vi "cRIO_ZNB_AMI_GLOBALES.vi"() -> ()   [LabVIEW 2017]
uses:
  RohdeSchwarz ZNB MeasConfig.ctl
  AMI MAGNET/Status AMI.ctl
  WEB Readings/Temperaturas Bluefors.ctl
  AMI MAGNET/commsControl.ctl
panel:
  in  "EN":bool
  in  "x":dbl min=-0.5 max=0.5 step=0.001 format="%.2f"
  in  "y":dbl min=-0.5 max=0.5 step=0.001 format="%.2f"
  out "ConfigX":T1={"connection ID"=refnum, "IP"="192.168.0.108", "Active Comm Interface"=0, "Serial Port"="", "Programmer Type"=0, "connection ID"=refnum, "output cluster"={"GPIB address"=22, "GPIB bus"=1}} {"Programmer Type" items=["Model 430", "Model 420"]; "Active Comm Interface" items=["TCP/IP (Model 430 Only)", "RS232", "IEEE488"]}
  out "ConfigY":T1={"connection ID"=refnum, "IP"="192.168.0.108", "Active Comm Interface"=0, "Serial Port"="", "Programmer Type"=0, "connection ID"=refnum, "output cluster"={"GPIB address"=22, "GPIB bus"=1}} {"Programmer Type" items=["Model 430", "Model 420"]; "Active Comm Interface" items=["TCP/IP (Model 430 Only)", "RS232", "IEEE488"]}
  out "ConfigZ":T1={"connection ID"=refnum, "IP"="192.168.0.108", "Active Comm Interface"=0, "Serial Port"="", "Programmer Type"=0, "connection ID"=refnum, "output cluster"={"GPIB address"=22, "GPIB bus"=1}} {"Programmer Type" items=["Model 430", "Model 420"]; "Active Comm Interface" items=["TCP/IP (Model 430 Only)", "RS232", "IEEE488"]}
  in  "Remote GO XYZ":bool
  out "F Stable":bool
  in  "FRemoteChange":bool
  out "Field Status":i32(ring) items=["MagnetUnknown"=0, "StablePersistent"=1, "WarmingSwitch"=2, "CoolingSwitch"=3, "StableDriven"=4, "Iterating"=5, "Charging"=6, "Discharging"=7, "CurrentError"=8, "MagnetFailure"=15]
  in  "MagneticField(T)":dbl
  in  "R_spField(T)":dbl=20.0
  in  "W_spField(T)":dbl
  in  "Rate(T/min)":dbl=0.1
  in  "SetpointB(T)":dbl
  in  "Electroiman(s)":dbl=0.5
  in  "ElectroimanEnable":bool=TRUE
  in  "stopElectroiman":bool
  in  "Remote DEMAG X":bool
  in  "Remote DEMAG Y":bool
  in  "Remote DEMAG Z":bool
  out "Z Stable":bool
  out "Y Stable":bool
  in  "BF RemoteChange":bool
  in  "url":string="http://192.168.0.101:5001/channel/measurement/latest"
  in  "Enable BF(T)":bool=TRUE
  in  "stopBluefors":bool
  out "BLUEFORS":T2 {"Canal 8" format="%.3f"; "Canal 7" format="%.3f"; "Canal 6" format="%.3f"; "Canal 5" format="%.3f"; "Canal 4" format="%.3f"; "Canal 3" format="%.3f"; "Canal 2" format="%.3f"; "Canal 1" format="%.3f"}
  in  "rampingMode X":u16(ring)=1 items=["RAMP", "PAUSE", "MANUAL UP", "MANUAL DOWN", "ZERO"]
  in  "rampingMode Y":u16(ring)=1 items=["RAMP", "PAUSE", "MANUAL UP", "MANUAL DOWN", "ZERO"]
  in  "rampingMode Z":u16(ring)=1 items=["RAMP", "PAUSE", "MANUAL UP", "MANUAL DOWN", "ZERO"]
  in  "stopMagneticField":bool
  in  "Remote SET Z":bool
  in  "Remote GO X":bool
  in  "Remote GO Y":bool
  in  "Remote SET X":bool
  in  "Remote SET Y":bool
  in  "Remote GO Z":bool
  out "X state":T3=1 items=["Unknown", "RAMPING to target field/current", "HOLDING at the target field/current", "PAUSED", "Ramping in MANUAL UP mode", "Ramping in MANUAL DOWN mode", "ZEROING CURRENT (in progress)", "Quench detected", "At ZERO current", "Heating persistent switch", "Cooling persistent switch", "External Rampdown active"]
  in  "Target X":dbl format="%.2f"
  in  "Rate X":dbl=0.1 format="%.2f"
  out "X field":dbl format="%.2f"
  out "Y state":T3=1 items=["Unknown", "RAMPING to target field/current", "HOLDING at the target field/current", "PAUSED", "Ramping in MANUAL UP mode", "Ramping in MANUAL DOWN mode", "ZEROING CURRENT (in progress)", "Quench detected", "At ZERO current", "Heating persistent switch", "Cooling persistent switch", "External Rampdown active"]
  in  "Target Y":dbl format="%.2f"
  in  "Rate Y":dbl=0.1 format="%.2f"
  out "Y field":dbl format="%.2f"
  out "Z state":T3=1 items=["Unknown", "RAMPING to target field/current", "HOLDING at the target field/current", "PAUSED", "Ramping in MANUAL UP mode", "Ramping in MANUAL DOWN mode", "ZEROING CURRENT (in progress)", "Quench detected", "At ZERO current", "Heating persistent switch", "Cooling persistent switch", "External Rampdown active"]
  in  "Target Z":dbl format="%.2f"
  in  "Rate Z":dbl=0.1 format="%.2f"
  out "Z field":dbl format="%.2f"
  out "Z ramping":bool
  out "Y ramping":bool
  out "X ramping":bool
  out "XY Graph":cluster{dbl[], dbl[]}(graph)
  out "VISA ENA3G":refnum<visa-resource-name>="GPIB0::17::INSTR"
  in  "ENA3G Config":T4={"Tiempo (sec)"=10.0, "Campo X (T)"=0.025, "Campo Y (T)"=10.0, "Campo Z (T)"=0.025, "Temperatura (K)"=0.025, "Start Frequency (Hz)"=100000.0, "Stop Frequency (Hz)"=1000000.0, "IF Bandwidth"=25.0, "Sweep time(s)"=25.0, "Meas Points"=201, "Power Level (0.0)"=-40.0} {"Campo Z (T)" format="%^.2e"; "Campo Y (T)" format="%^.2e"; "Sweep time(s)" format="%^.2g"; "Temperatura (K)" format="%^.2e"; "Campo X (T)" format="%^.2e"; "Tiempo (sec)" format="%^.2g"; "Start Frequency (Hz)" format="%^.2e"; "IF Bandwidth" format="%^.2e"; "Power Level (0.0)" format="%^.2g"}
  in  "VRemoteChange":bool
  out "Voltage Status":i32(ring) items=["VoltageUnknown", "Stable", "Tracking"]
  out "V Stable":bool
  in  "RampaVolt(V)":dbl
  in  "R_spVolt(V)":dbl=20.0
  in  "W_spVolt(V)":dbl
  in  "Rate(V/min)":dbl=0.1
  in  "SetpointV(V)":dbl
  in  "RampaVolt(s)":dbl=0.5
  in  "RampaVoltajeEnable":bool=TRUE
  in  "stopRampaVolt":bool
  in  "FieldCalPath":path=path "C:/Users/pemar/Documents/LabVIEW Data/XImanCalibre.txt"
  in  "TempCalPath":path=path "C:/Users/pemar/Documents/LabVIEW Data/X71548_InterpNew.txt"
  in  "TRemoteChange":bool
  out "DataPath":path
  out "Total Comandos":i32
  out "Comando actual":i32
  out "TotalSequence":string[](array[string])
  in  "stop":bool
  out "Temperature Status":i32(ring) items=["TemperatureUnknown", "Stable", "Tracking", "Near"]
  out "X Stable":bool
  out "T Stable":bool
  in  "R_spTemp(K)":dbl=20.0
  in  "W_spTemp(K)":dbl
  in  "VISA LakeShore":refnum<visa-resource-name>="COM3"
  in  "SaveData":bool=TRUE
  in  "Rate(K/min)":dbl=20.0
  in  "SetpointT(K)":dbl
  in  "Temperatura(K)":dbl
  in  "LakeShoreEnable":bool=TRUE
  in  "LakeShore(s)":dbl=0.5
  in  "stopLakeShore":bool
  in  "Estado":bool=TRUE
  in  "InitGraph":bool=TRUE
  in  "AMI Enable":bool=TRUE
  # "Z axis"
  # "Y axis"
  # "X axis"
  # "STATUS"
  # "STATUS"
  # "STATUS"
  # "SETTINGS"
  # "SETTINGS"
  # "SETTINGS"
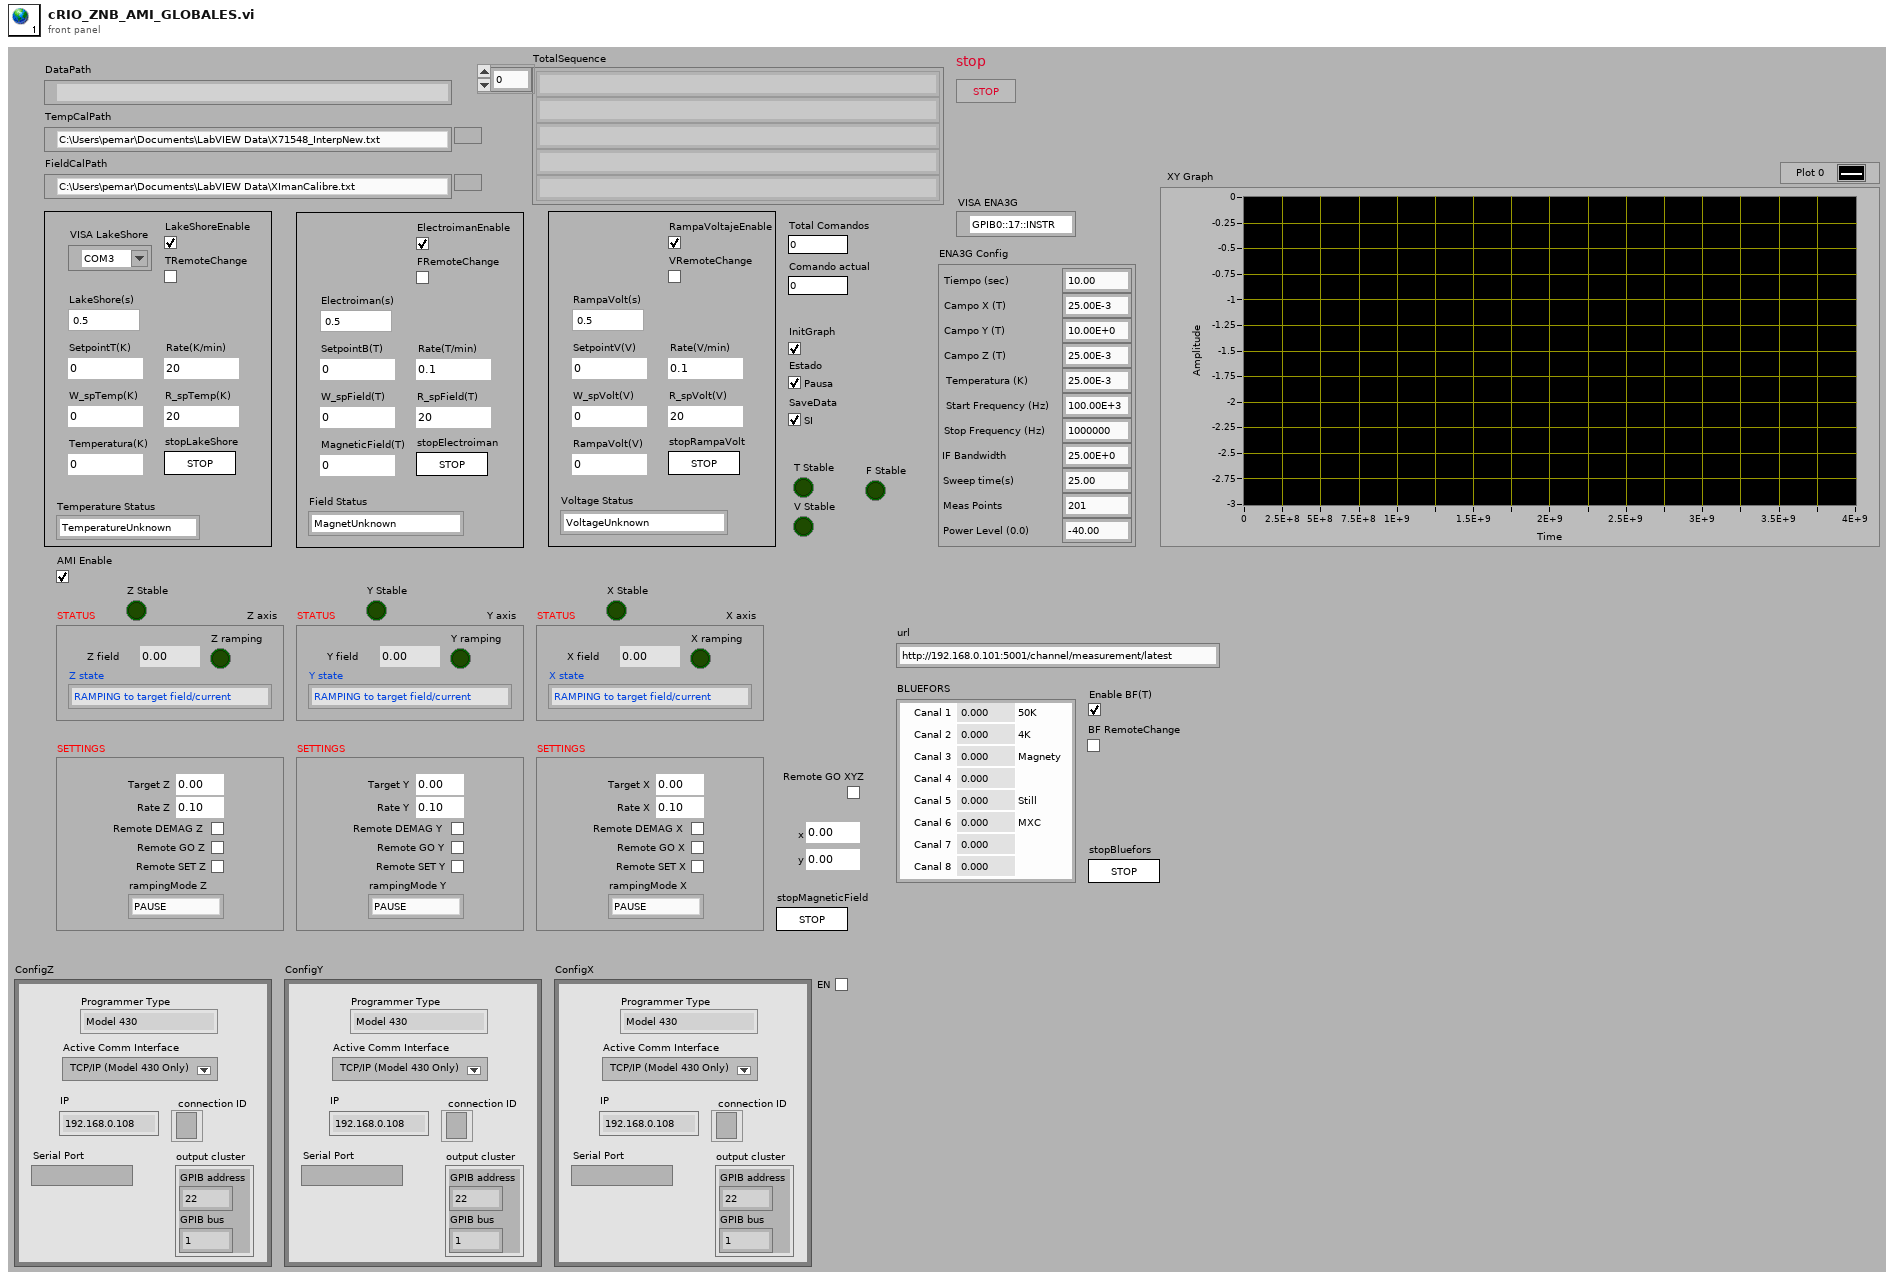
[diagram p1: front panel]
types:
  T1 = typedef "commsControl.ctl" = cluster{"connection ID":refnum<k5>, "IP":string, "Active Comm Interface":u16, "Serial Port":refnum<visa-resource-name>, "Programmer Type":u16, "connection ID":refnum<k5>, "output cluster":cluster{"GPIB address":i16, "GPIB bus":i16}}
  T2 = typedef "Temperaturas Bluefors.ctl" = cluster{"Canal 1":dbl, "Canal 2":dbl, "Canal 3":dbl, "Canal 4":dbl, "Canal 5":dbl, "Canal 6":dbl, "Canal 7":dbl, "Canal 8":dbl}
  T3 = typedef "Status AMI.ctl" = u16
  T4 = typedef "RohdeSchwarz ZNB MeasConfig.ctl" = cluster{"Tiempo (sec)":dbl, "Campo X (T)":dbl, "Campo Y (T)":dbl, "Campo Z (T)":dbl, "Temperatura (K)":dbl, "Start Frequency (Hz)":dbl, "Stop Frequency (Hz)":dbl, "IF Bandwidth":dbl, "Sweep time(s)":dbl, "Meas Points":i32, "Power Level (0.0)":dbl}
diagram:
